vi "Search HPS Network.vi"(0 "reference in":refnum<class "HPS-17000-PowerModule.lvclass">, 5 "Controller TSN IP":string, 7 "Network Search Completed":refnum<user-event>, 11 "Error In":errorcluster) -> (4 "reference out":refnum<class "HPS-17000-PowerModule.lvclass">, 15 "Error Out":errorcluster)   [LabVIEW 2023, in "HPS-17000-PowerModule.lvlib" / "HPS-17000-PowerModule.lvclass"]
uses:
  HPS-17000-PowerModule.lvclass
  HPS-17000-PowerModule.lvclass/HPS-17000-PowerModule.ctl
  <instrlib>/HPS-17000/HPS-17000.lvclass
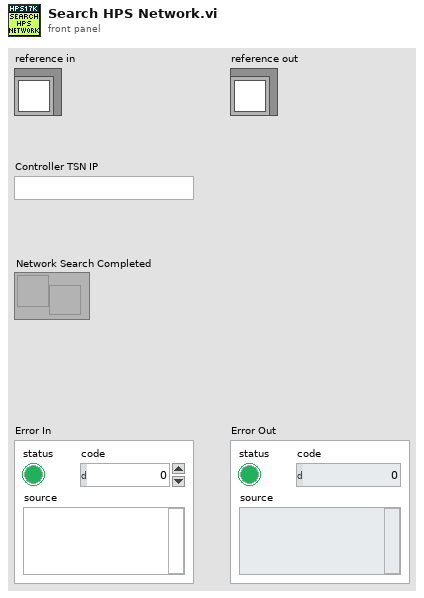
[diagram p1: front panel]
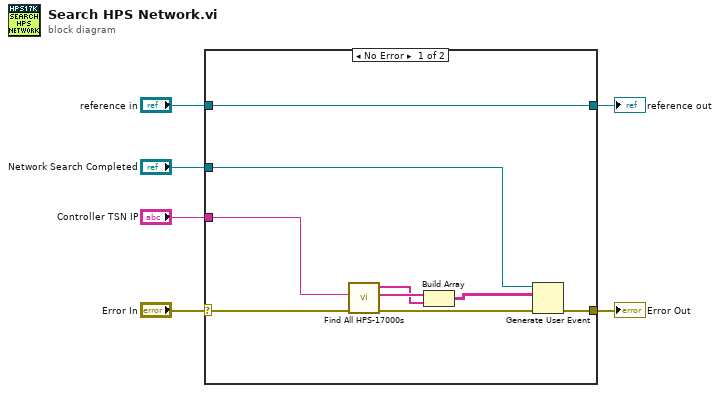
[diagram p0: block diagram]
diagram:
  n1 = case shown="No Error" "Error In" {
    selector: "Error In" -> [w7 w17]
    tunnel: [w15 w17] -> w5
    tunnel: [w8 w16] -> w3
    tunnel: "reference in" -> [w8 w16]
    tunnel: "Network Search Completed" -> [w14 _]
    tunnel: "Controller TSN IP" -> [w13 _]
    frame No Error {
      n2 = call <instrlib>:"Find All HPS-17000s.vi"("error in"=w7, "controller TSN IP"=w13) -> ("error out"=w12:errorcluster, "HPS-17000 IPs"=w11:string[], "HPS-17000 names"=w10:string[])  [unwired: 7 in]
      n3 = Build Array(w11, w10) -> (w9:string[][])
      n4 = Generate User Event(user event=w14, event data cluster=w9, error in=w12) -> (error out=w15:errorcluster)  [unwired: 1 in, 1 out]
    }
    frame Error {
    }
  }
  "Error Out" <- w5
  "reference out" <- w3
